vi "VSSDecodeFIRASimBall.vi"(8 "error in (no error)":errorcluster, 9 "TimeStamp":timestamp, 11 "Frame":u8[](array[numeric])) -> (0 "error out":errorcluster, 2 "Robots":u8[](array[numeric]), 3 "Balls out":T1[](array[typedef]))   [LabVIEW 2018]
uses:
  Controls/SSL Detection Ball.ctl
  <vilib>/Analysis/Matrix/Datatypes/RealMatrix.ctl
  <vilib>/Analysis/Matrix/NI_Matrix.lvlib
panel:
  in  "Ball":T1
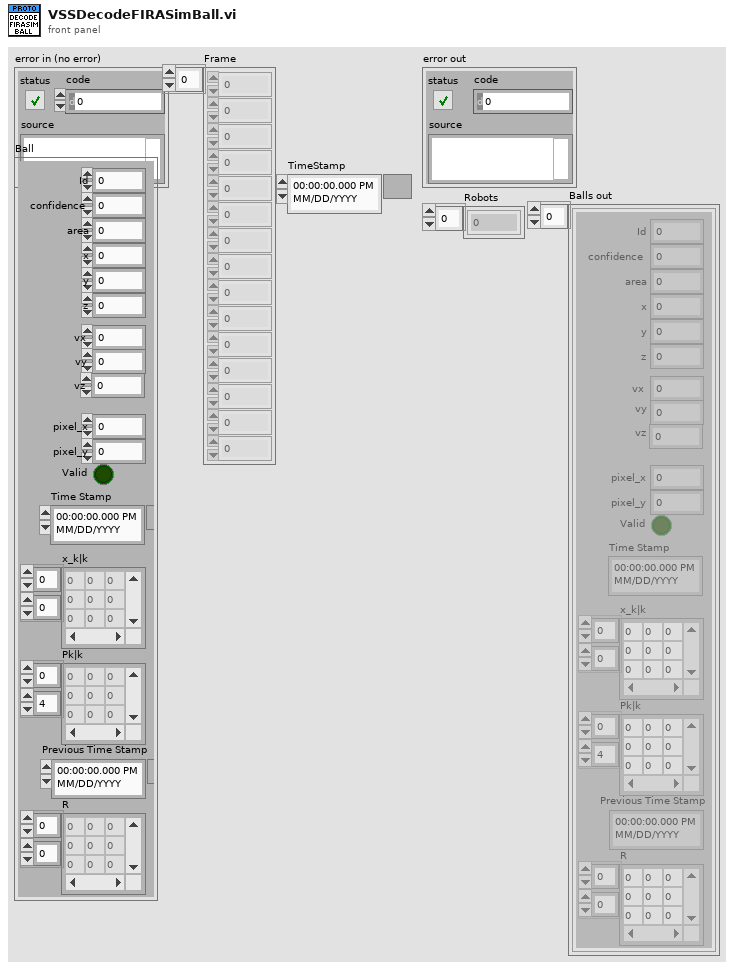
[diagram p1: front panel]
types:
  T1 = typedef "SSL Detection Ball.ctl" = cluster{"x":sgl, "area":u32, "confidence":sgl, "y":sgl, "z":sgl, "pixel_x":sgl, "pixel_y":sgl, "Valid":bool, "Time Stamp":timestamp, "x_k|k":T2, "Pk|k":T2, "Id":u32, "Previous Time Stamp":timestamp, "R":T2, " vx":sgl, "vy":dbl, "vz":dbl}
  T2 = typedef "NI_Matrix.lvlib/RealMatrix.ctl" = dbl[][]
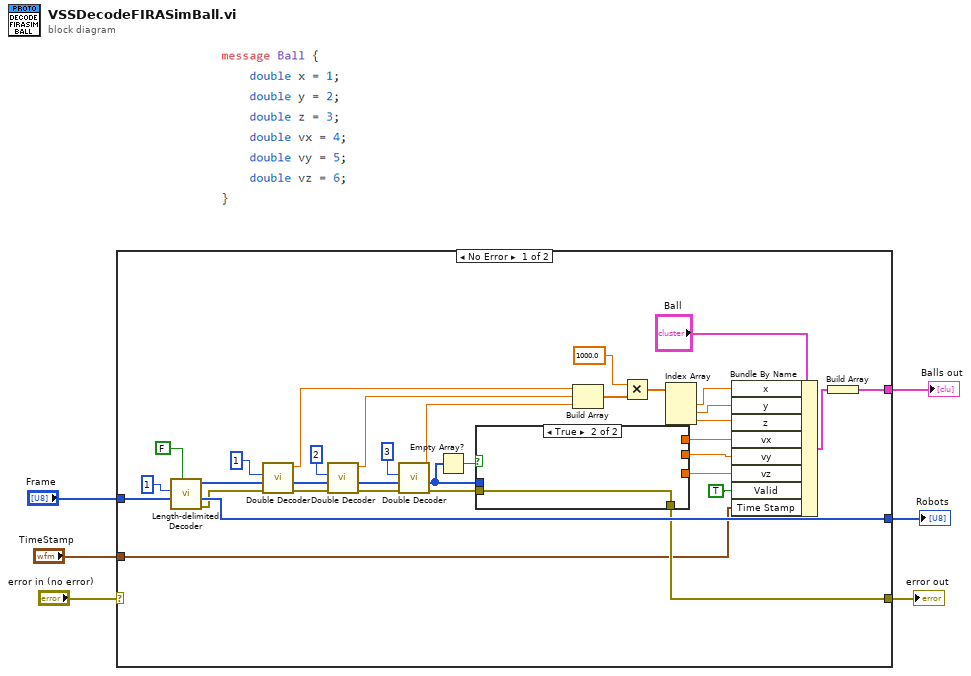
[diagram p0: block diagram]
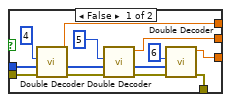
[diagram p2: hidden frame]
diagram:
  n1 = case shown="No Error" "error in (no error)" {
    selector: "error in (no error)" -> [_ w55]
    tunnel: [w25 w55] -> w5
    tunnel: "Frame" -> [w40 _]
    tunnel: [w38 _] -> w3
    tunnel: [w23 _] -> w1
    tunnel: "TimeStamp" -> [w24 _]
    frame No Error {
      n2 = call "Length-delimited Decoder.vi"("Optional"=FALSE, "Array"=w40, "Key"=1) -> ("error out"=w28:errorcluster, "array w/ subset deleted"=w38:u8[], "Length-delimited"=w37:u8[])  [unwired: 5 in, 1 out]
      n3 = call "Double Decoder.vi"("error in (no error)"=w28, "Array"=w37, "Key"=1) -> ("error out"=w29:errorcluster, "array w/ subset deleted"=w36:u8[], "Double"=w21:dbl)  [unwired: 5 in, 1 out]
      n4 = call "Double Decoder.vi"("error in (no error)"=w29, "Array"=w36, "Key"=2) -> ("error out"=w27:errorcluster, "array w/ subset deleted"=w35:u8[], "Double"=w20:dbl)  [unwired: 5 in, 1 out]
      n5 = call "Double Decoder.vi"("error in (no error)"=w27, "Array"=w35, "Key"=3) -> ("error out"=w26:errorcluster, "array w/ subset deleted"=w7:u8[], "Double"=w19:dbl)  [unwired: 5 in, 1 out]
      n6 = Empty Array?(array=w7) -> (empty?=w8:bool)
      n7 = case shown="True" w8 {
        tunnel: w7 -> [w53 _]
        tunnel: w26 -> [w47 w54]
        tunnel: [w44 w54] -> w25
        tunnel: [w43 _] -> w12
        tunnel: [w42 _] -> w11
        tunnel: [w41 _] -> w10
        frame False {
          n8 = call "Double Decoder.vi"("error in (no error)"=w47, "Array"=w53, "Key"=4) -> ("error out"=w46:errorcluster, "array w/ subset deleted"=w52:u8[], "Double"=w43:dbl)  [unwired: 5 in, 1 out]
          n9 = call "Double Decoder.vi"("error in (no error)"=w46, "Array"=w52, "Key"=5) -> ("error out"=w45:errorcluster, "array w/ subset deleted"=w51:u8[], "Double"=w42:dbl)  [unwired: 5 in, 1 out]
          n10 = call "Double Decoder.vi"("error in (no error)"=w45, "Array"=w51, "Key"=6) -> ("error out"=w44:errorcluster, "Double"=w41:dbl)  [unwired: 5 in, 2 out]
        }
        frame True {
        }
      }
      n11 = Build Array(w21, w20, w19) -> (w18:dbl[])
      n12 = Multiply(x=1000.0, y=w18) -> (x*y=w16:dbl[])
      n13 = Index Array(array=w16) -> (element #1=w15:dbl, element #2=w14:dbl, element #3=w13:dbl)  [unwired: 3 in]
      n14 = Bundle By Name(cluster="Ball", "x"=w15, "y"=w14, "z"=w13, "vx"=w12, "vy"=w11, "vz"=w10, "Valid"=TRUE, "Time Stamp"=w24) -> (w22:T1)
      n15 = Build Array(w22) -> (w23:T1[])
    }
    frame Error {
    }
  }
  "error out" <- w5
  "Robots" <- w3
  "Balls out" <- w1
